vi "Configure Device.vi"(8 "error in":errorcluster, 11 "CnPt in":refnum<class "CnPt.lvclass">) -> (0 "error out":errorcluster, 3 "CnPt out":refnum<class "CnPt.lvclass">, 4 "SP":dbl, 5 "Settable?":bool)   [LabVIEW 2015, in "CnPt.lvclass"]
uses:
  CnPt.lvclass
  <vilib>/MSR Consulting, LLC/General Reuse/Session APIs/Serial/Typedefs/Session Handle.ctl
  <vilib>/MSR Consulting, LLC/General Reuse/Session APIs/Serial/Serial Session.lvclass
  Mode.ctl
  <vilib>/MSR Consulting, LLC/Devices/Configurable Device/Configurable Device.lvclass/Configurable Device.ctl
  <vilib>/MSR Consulting, LLC/General Reuse/Session APIs/File Access/Config Data/Config Data.lvclass/Config Data.ctl
  CnPt.lvclass/CnPt.ctl
  <vilib>/MSR Consulting, LLC/Devices/Configurable Device/Read Handle.vi
  <vilib>/MSR Consulting, LLC/Devices/Configurable Device/Accessors/Read Config Section.vi
  <vilib>/MSR Consulting, LLC/General Reuse/Session APIs/File Access/Config Data/Accessors/Read Ref.vi
  Accessors/Write Serial Handle.vi
  Write Alarm Range.vi
  Write Run_.vi
  <vilib>/Utility/config.llb/Read Key (Double).vi
  <vilib>/Utility/config.llb/Read Key (Boolean).vi
  Set Temperature.vi
  Set Mode.vi
  <vilib>/MSR Consulting, LLC/General Reuse/Session APIs/File Access/Config Data/Config Data.lvclass
  <vilib>/MSR Consulting, LLC/General Reuse/Session APIs/_Session Fwk/Session - Root.lvclass
  <vilib>/Utility/config.llb/NI_LVConfig.lvlib
panel:
  in  "Session":string="TSI 3550"
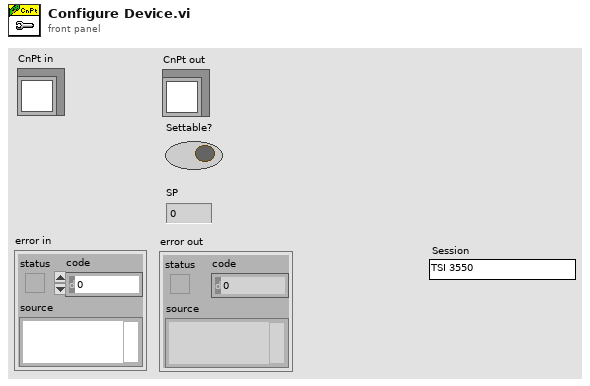
[diagram p1: front panel]
types:
  T1 = typedef "CnPt.lvclass/Mode.ctl" = u16
  T2 = typedef "Serial Session.lvclass/Session Handle.ctl" = refnum<data-value>
  T3 = typedef "Config Data.lvclass/Config Session.ctl" = refnum<data-value>
  T4 = typedef "NI_LVConfig.lvlib/Config Data RefNum.ctl" = refnum<k1>
  T5 = typedef "Session - Root.lvclass/Session Handle.ctl" = refnum<data-value>
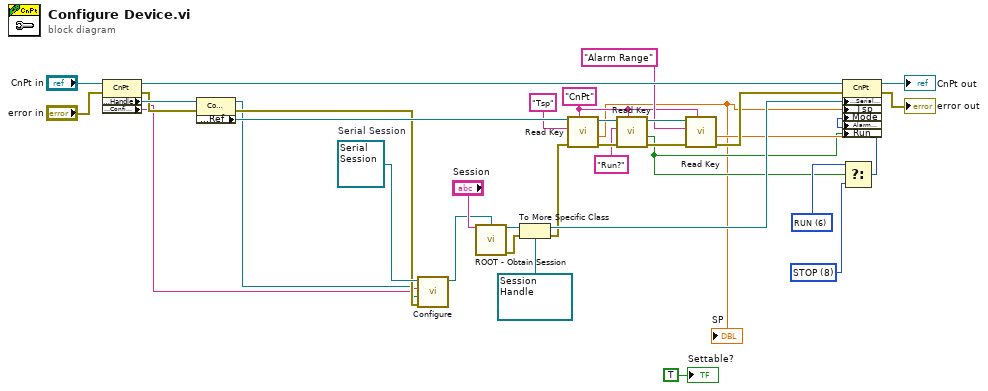
[diagram p0: block diagram]
diagram:
  w7 = refnum<class "Serial Session.lvclass"> refnum  # Serial Session
  w16 = T1 6 items=["RUN"=6, "STANDBY"=7, "STOP"=8, "PAUSE"=9] ("Mode")
  w17 = T1 8 items=["RUN"=6, "STANDBY"=7, "STOP"=8, "PAUSE"=9] ("Mode")
  w9 = "CnPt" ("Section Name")
  n1 = property class="CnPt"(reference="CnPt in", error in="error in") -> (reference out=w28:refnum<class "CnPt.lvclass">, error out=w32:errorcluster, "Accessors:Handle"=w33:T3, "Accessors:Config Section"=w3:string)
  n2 = property class="Config Data"(reference=w33, error in=w32) -> (reference out=w4:T3, error out=w5:errorcluster, "Accessors:Ref"=w30:T4)
  n3 = call <vilib>:"Configure.vi"("error in"=w5, "Config Handle"=w4, "section"=w3, "Serial Session in"=w7) -> ("Serial Session out"=w6:refnum<class "Serial Session.lvclass">)  [unwired: 6 in, 1 out]
  n4 = call <vilib>:"ROOT - Obtain Session.vi"("Session Name ()"="Session", "OBJ - Session"=w6) -> ("Session Handle"=w25:T5, "error out"=w22:errorcluster)  [unwired: 11 in, 1 out]
  n5 = To More Specific Class(target class=T2 refnum ("Serial Handle"), reference=w25, error in=w22) -> (specific class reference=w23:T2, error out=w21:errorcluster)
  n6 = call-poly <vilib>:"Read Key.vi"("section"=w9, "error in (no error)"=w21, "key"="Tsp", "refnum"=w30) -> ("error out"=w19:errorcluster, "value"=w1:dbl, "refnum out"=w20:T4)  [unwired: 4 in, 1 out]
  "SP" <- w1
  n7 = call-poly <vilib>:"Read Key.vi"("section"=w9, "error in (no error)"=w19, "key"="Run?", "refnum"=w20) -> ("error out"=w14:errorcluster, "value"=w8:bool, "refnum out"=w13:T4)  [unwired: 4 in, 1 out]
  n8 = call-poly <vilib>:"Read Key.vi"("section"=w9, "error in (no error)"=w14, "key"="Alarm Range", "refnum"=w13) -> ("error out"=w12:errorcluster, "value"=w10:dbl)  [unwired: 4 in, 2 out]
  n9 = Select(t=w16, s=w8, f=w17) -> (s? t:f=w15:T1)
  n10 = property class="CnPt"(reference=w28, error in=w12, "Accessors:Serial Handle"=w23, "Tsp"=w1, "Mode"=w15, "Alarm Range"=w10, "Run_"=w8) -> (reference out=→"CnPt out":refnum<class "CnPt.lvclass">, error out=→"error out":errorcluster)
  "Settable?" <- TRUE ("Settable?")
